vi "Stop Acquisition.vi"(8 "error in (no error)":errorcluster, 10 "report in":refnum<class "NI_report.lvclass">, 11 "Hardware Resources in":T1={"Test Setting"={"Test_Num"=0, "Test_ID"=0, "Proc_ID"=0, "Max Force"=0.0, "User"="", "SN"="", "Date"=""}, "Measurements"=[[""]], "LOG REF"=refnum, "Report Template"=path "", "Save Report path"=path "", "Data File Path"=path "", "Popup Dialog"=FALSE}) -> (0 "error out":errorcluster)   [LabVIEW 2020, in "Report.lvlib"]
doc: "Stops the acquisition."
uses:
  Report.lvlib
  REP Configuration.ctl
  Test Setting.ctl
  <vilib>/Utility/NIReport.llb/NI_report.lvclass
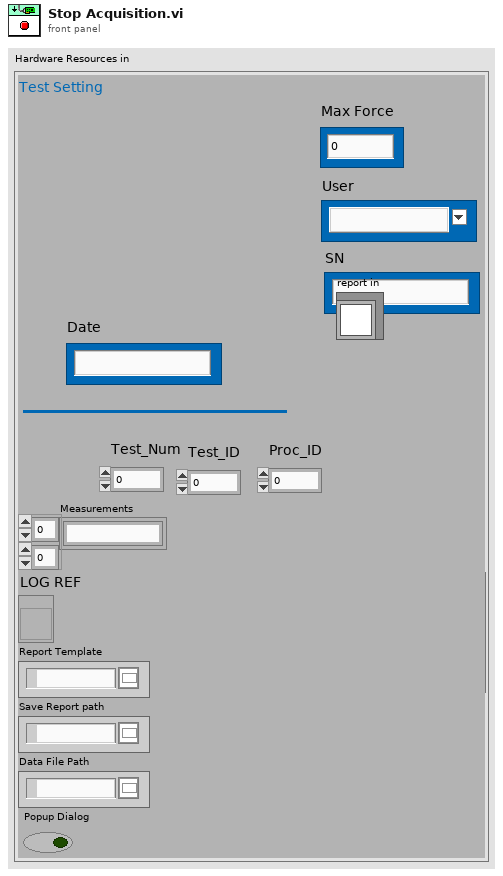
[diagram p1: front panel]
types:
  T1 = typedef "Report.lvlib/REP Configuration.ctl" = cluster{"Test Setting":T2, "Measurements":string[][], "LOG REF":refnum<vi>, "Report Template":path, "Save Report path":path, "Data File Path":path, "Popup Dialog":bool}
  T2 = typedef "Report.lvlib/Test Setting.ctl" = cluster{"Test_Num":i32, "Test_ID":i32, "Proc_ID":i32, "Max Force":dbl, "User":string, "SN":string, "Date":string}
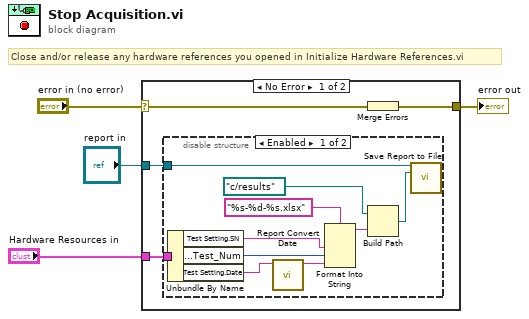
[diagram p0: block diagram]
diagram:
  # "Close and/or release any hardware references you opened in Initialize Hardware References.vi"
  n1 = case shown="No Error" "error in (no error)" {
    selector: "error in (no error)" -> [w7 w19]
    tunnel: [w8 w19] -> w3
    tunnel: "Hardware Resources in" -> [w6 _]
    tunnel: "report in" -> [w5 _]
    frame No Error {
      n2 = disable-structure shown="Enabled" {
        disable-tunnel: w6 -> [w18 _]
        disable-tunnel: w5 -> [w13 _]
        frame Enabled {
          n3 = Unbundle By Name(w18) -> ("Test Setting.SN"=w12:string, "Test Setting.Test_Num"=w11:i32, "Test Setting.Date"=w10:string)
          n4 = call "Report Convert Date.vi"("Date"=w10) -> ("result string"=w9:string)  [unwired: 10 in]
          n5 = Format Into String(format string="%s-%d-%s.xlsx", w12, w11, w9) -> (resulting string=w16:string)  [unwired: 2 in, 1 out]
          n6 = Build Path(base path=path "c:/results" ("report file path"), name or relative path=w16) -> (appended path=w14:path)
          n7 = call-dynamic "Save Report to File.vi"("report in"=w13, "report file path"=w14) -> ()  [unwired: 12 in, 2 out]
        }
        frame Disabled {
        }
      }
      n8 = Merge Errors(w7) -> (w8:errorcluster)
    }
    frame Error {
    }
  }
  "error out" <- w3
